vi "Run.vi"(8 "error in (no error)":errorcluster, 10 "Test":refnum<class "Test.lvclass">, 11 "TestResultMock in":refnum<class "TestResultMock.lvclass">) -> (0 "error out":errorcluster, 2 "Test out":refnum<class "Test.lvclass">, 3 "TestResultMock out":refnum<class "TestResultMock.lvclass">)   [LabVIEW 2017, in "TestSuiteTest.lvlib" / "Support.lvlib" / "TestResultMock.lvclass"]
doc: "Runs a <B>TestCase</B>."
uses:
  TestResultMock.lvclass
  Test/Test.lvclass
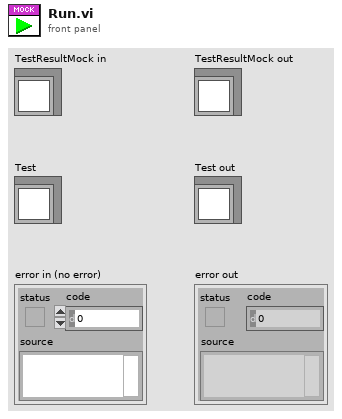
[diagram p1: front panel]
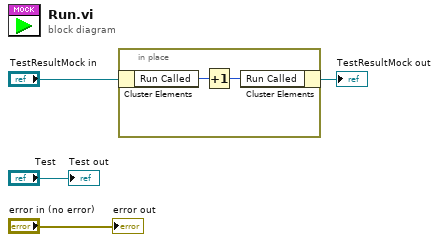
[diagram p0: block diagram]
diagram:
  n1 = in-place {
    n2 = in-place-cluster #1("TestResultMock in") -> ("Run Called"=w6:i32)
    n3 = Increment(x=w6) -> (x+1=w5:i32)
    n4 = in-place-cluster #1("Run Called"=w5) -> (→"TestResultMock out":refnum<class "TestResultMock.lvclass">)
  }
  "error out" <- "error in (no error)"
  "Test out" <- "Test"
